vi "Core.vi"(11 "Instrument in":refnum<class "Instrument.lvclass">) -> ()   [LabVIEW 2014, in "Instrument.lvclass"]
doc: "The Core is a reentrant template for basic operation of the instrument. This sets the default mode to Acquire. Configuration is done outside of the basic operation and commands are sent via a command queue using a command pattern."
uses:
  Instrument.lvclass
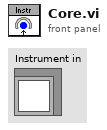
[diagram p1: front panel]
types:
  T1 = typedef "Instrument.lvclass/state.ctl" = enum8{"Configure", "Acquire", "Wait", "Quit", "Handle Error", "NOOP"}
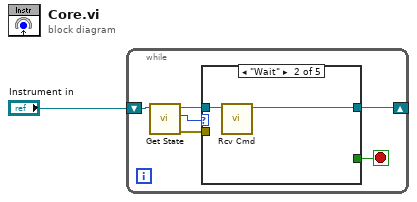
[diagram p0: block diagram]
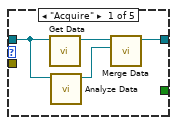
[diagram p2: hidden frame]
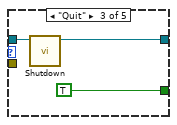
[diagram p3: hidden frame]
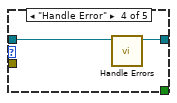
[diagram p4: hidden frame]
diagram:
  n1 = while {
    shift-right: [w3] -> _
    shift-left: "Instrument in" -> [w4]
    stop <- w6 stop-if-true
    n2 = call "Get State.vi"("Instrument in"=w4) -> ("error out"=w2:errorcluster, "default state"=w7:T1, "Instrument out"=w5:refnum<class "Instrument.lvclass">)  [unwired: 8 in]
    n3 = case shown="\"Wait\"" w7 {
      tunnel: [_ _ TRUE _ _] -> w6
      tunnel: w5 -> [w11 w13 w15 w18 w19]
      tunnel: [w10 w12 w14 w17 w19] -> w3
      tunnel: w2 -> [_ _ _ _ _]
      frame "Acquire" {
        n4 = call-dynamic "Get Data.vi"("Instrument in"=w11) -> ("Instrument out"=w9:refnum<class "Instrument.lvclass">)  [unwired: 9 in, 1 out]
        n5 = call-dynamic "Analyze Data.vi"("Instrument in"=w11) -> ("Instrument out"=w8:refnum<class "Instrument.lvclass">)  [unwired: 9 in, 1 out]
        n6 = call-dynamic "Merge Data.vi"("Analyzed"=w8, "Acquired"=w9) -> ("Instrument out"=w10:refnum<class "Instrument.lvclass">)  [unwired: 8 in, 1 out]
      }
      frame "Wait" {
        n7 = call-dynamic "Rcv Cmd.vi"("Instrument in"=w13) -> ("Instrument out"=w12:refnum<class "Instrument.lvclass">)  [unwired: 9 in, 1 out]
      }
      frame "Quit" {
        n8 = call-dynamic "Shutdown.vi"("Instrument in"=w15) -> ("Instrument out"=w14:refnum<class "Instrument.lvclass">)  [unwired: 9 in, 1 out]
      }
      frame "Handle Error" {
        n9 = call-dynamic "Handle Errors.vi"("Instrument in"=w18) -> ("Instrument out"=w17:refnum<class "Instrument.lvclass">)  [unwired: 8 in, 2 out]
      }
      frame "NOOP", Default {
      }
    }
  }
